vi "诊断标定3 - 副本.vi"(8 "CAN端口":u16(ring), 9 "设备索引号":u16(ring), 10 "CAN卡类型":u32(ring)=21) -> ()   [LabVIEW 2013] (continued)
                          n766 = Concatenate Strings("读取错误，代码： " ("字符串"), "0x" ("字符串"), w1225) -> (w1223:string)
                          n767 = One Button Dialog(message=w1223, button name ("OK")="是" ("按钮名称（“确定”）")) -> ()  [unwired: 1 out]
                        }
                      }
                      n768 = local write "消除"(FALSE ("消除")) -> ()
                      n769 = global write "EV05全局变量1.vi" "流控帧 2"(FALSE ("流控帧 2")) -> ()
                      n770 = local write "控制1"(FALSE ("控制1")) -> ()
                      n771 = global write "EV05全局变量1.vi" "写入超时"(TRUE ("写入超时")) -> ()
                    }
                  }
                }
              }
            }
          }
        }
      }
      frame Error {
      }
    }
  }
  n772 = while {
    tunnel: w36 -> [w1240]
    tunnel: w35 -> [w1239]
    tunnel: [w1238] -> w34
    tunnel: [w1237] -> w33
    tunnel: w23 -> [_]
    tunnel: w20 -> [_]
    stop <- w1236 stop-if-true
    n773 = event shown="[16] \"主板选项\": 鼠标按下" {
      selector: _ -> [_ _ _ _ _ _ _ _ _ _ _ _ _ _ _ _ _ _ _ _ _ _ _ _ _ _ _ _ _ _ _ _ _ _ _ _ _ _ _ _ _ _ _ _ _ _ _ _ _ _ _ _ _]
      dyn-events: _ -> [_ _ _ _ _ _ _ _ _ _ _ _ _ _ _ _ _ _ _ _ _ _ _ _ _ _ _ _ _ _ _ _ _ _ _ _ _ _ _ _ _ _ _ _ _ _ _ _ _ _ _ _ _]
      timeout: 200 -> [_ _ _ _ _ _ _ _ _ _ _ _ _ _ _ _ _ _ _ _ _ _ _ _ _ _ _ _ _ _ _ _ _ _ _ _ _ _ _ _ _ _ _ _ _ _ _ _ _ _ _ _ _]
      tunnel: [_ w1243 w1283 _ _ _ _ _ _ _ _ _ _ _ _ _ _ _ _ _ _ _ _ _ _ _ _ _ _ _ _ _ _ _ _ _ _ _ _ _ _ _ _ _ _ _ _ _ _ _ _ _ _] -> w1235
      tunnel: w1240 -> [w1242 w1246 w1282 _ w1323 w1334 w1345 w1356 w1367 w1378 w1389 w1400 w1411 w1422 w1433 w1444 w1460 w1998 w2420 w2445 w2473 w2576 w2649 w2662 w2672 w2718 _ _ w2768 w2835 w2902 w2969 w3036 w3103 w3170 w3238 w3306 w3373 w3440 w3510 w3521 w3560 w3600 w3640 w3680 w3718 w3778 w3813 w3849 w3882 w3952 w3985 w4018]
      tunnel: w1239 -> [w1241 w1245 w1281 _ w1322 w1333 w1344 w1355 w1366 w1377 w1388 w1399 w1410 w1421 w1432 w1443 w1459 w1997 w2419 w2444 w2472 w2575 w2647 w2660 w2671 w2717 _ _ w2767 w2834 w2901 w2968 w3035 w3102 w3169 w3237 w3305 w3372 w3439 w3508 w3520 w3559 w3599 w3639 w3679 w3717 w3777 w3812 w3848 w3881 w3951 w3984 w4017]
      tunnel: [w1242 w1246 w1282 _ w1323 w1334 w1345 w1356 w1367 w1378 w1389 w1400 w1411 w1422 w1433 w1444 w1460 w1998 w2420 w2445 w2473 w2576 w2648 w2661 w2672 w2718 _ _ w2768 w2835 w2902 w2969 w3036 w3103 w3170 w3238 w3306 w3373 w3440 w3509 w3519 w3558 w3598 w3638 w3678 w3718 w3776 w3811 w3847 w3880 w3950 w3983 w4016] -> w1238
      tunnel: [w1241 w1245 w1281 _ w1322 w1333 w1344 w1355 w1366 w1377 w1388 w1399 w1410 w1421 w1432 w1443 w1459 w1997 w2419 w2444 w2472 w2575 w2646 w2659 w2671 w2717 _ _ w2767 w2834 w2901 w2968 w3035 w3102 w3169 w3237 w3305 w3372 w3439 w3507 w3518 w3557 w3597 w3637 w3677 w3717 w3775 w3810 w3846 w3879 w3949 w3982 w4015] -> w1237
      tunnel: [_ _ _ _ _ _ _ _ _ _ _ _ _ _ _ _ _ _ _ _ _ _ _ _ _ _ _ _ _ _ _ _ _ _ _ _ _ _ _ _ w3518 w3557 w3597 w3637 w3677 _ w3775 w3810 w3846 w3879 w3949 w3982 w4015] -> w1234
      event Timeout {
        n774 = event-data() -> ()  [unwired: 3 out]
      }
      event "停止": Value Change {
        n775 = event-data() -> ("NewVal"=w1244:bool)  [unwired: 5 out]
        n776 = stacked-sequence {
          tunnel: w1244 -> [w1263 _]
          tunnel: [w1263 _] -> w1243
          frame #0 {
            n777 = global read "配置文件全局.vi" "诊断标定读取地址"() -> (w1247:path)
            n778 = call <vilib>:"Application Directory.vi"() -> ("Application Directory"=w1257:path)
            n779 = property class="VI"("FP.State"=T24."Hidden" ("前面板窗口:状态")) -> (reference out=w1259:refnum<vi>, error out=w1258:errorcluster)  [unwired: 2 in]
            n780 = Build Path(base path=w1257, name or relative path="config.ini" ("名称或相对路径")) -> (appended path=w1255:path)
            n781 = call <vilib>:"Open Config Data.vi"("configuration file path"=w1255) -> ("error out"=w1252:errorcluster, "refnum"=w1254:T25)  [unwired: 8 in, 1 out]
            n782 = local write "停止"(TRUE ("停止")) -> ()
            n783 = property class="VI"(reference=w1259, error in=w1258, "Front Panel.Open"=FALSE ("前面板窗口:打开")) -> ()  [unwired: 2 out]
            n784 = call-poly <vilib>:"Write Key.vi"("section"="总信息", "error in (no error)"=w1252, "value"=w1247, "key"="诊断标定读取地址" ("section"), "refnum"=w1254) -> ("error out"=w1251:errorcluster, "refnum out"=w1250:T25)  [unwired: 4 in, 1 out]
            n785 = call <vilib>:"Close Config Data.vi"("error in (no error)"=w1251, "refnum"=w1250) -> ("error out"=w1249:errorcluster)  [unwired: 8 in, 1 out]
            n786 = call <vilib>:"Clear Errors.vi"("error in (no error)"=w1249) -> ()  [unwired: 6 in, 1 out]
          }
          frame #1 {
            n787 = disable-structure shown="禁用" {
              frame Disabled {
                n788 = local read "设备索引号"() -> (w1269:u16)
                n789 = local read "CAN卡类型"() -> (w1270:u32)
                n790 = local read "CAN端口"() -> (w1268:u16)
                n791 = Build Array(7) -> (w1265:i32[])
                n792 = call "transmit-8.6.vi"("can卡类型"=w1270, "设备索引号"=w1269, "CAN端口"=w1268, "ID"=418398080, "SendType"=u8 0, "Data"=w1265) -> ()  [unwired: 3 in, 11 out]
              }
              frame Enabled {
                w1277 = u8 0 items=["Normal", "Listen Only"] ("工作方式")
                w1276 = u8 1 items=["Dual Filter", "Single Filter"] ("滤波方式")
                n793 = local read "设备索引号"() -> (w1272:u16)
                n794 = local read "CAN卡类型"() -> (w1271:u32)
                n795 = local read "CAN端口"() -> (w1273:u16)
                n796 = call "CAN_Init-8.6.vi"("CAN卡类型"=w1271, "设备索引号"=w1272, "CAN端口"=w1273, "操作类型"=enum16{"初始化CAN", "关闭CAN"}."初始化CAN", "滤波方式"=w1276, "Accept Code"=u32 0, "簇"=T21 {"打开CAN"=FALSE, "初始化CAN"=TRUE, "开始CAN"=TRUE, "重启"=FALSE, "关闭CAN"=FALSE}, "Mask Code"=u32 4294967295 ("Accept Code"), "工作方式"=w1277, "是否滤波"=FALSE) -> ()  [unwired: 4 in, 6 out]
              }
            }
          }
        }
      }
      event Panel Close? {
        n797 = event-data() -> ()  [unwired: 5 out]
        n798 = stacked-sequence {
          tunnel: [w1296 _] -> w1283
          frame #0 {
            w1296 = TRUE ("前面板窗口:打开")
            n799 = global read "配置文件全局.vi" "诊断标定读取地址"() -> (w1285:path)
            n800 = call <vilib>:"Application Directory.vi"() -> ("Application Directory"=w1295:path)
            n801 = property class="VI"("FP.State"=T24."Hidden" ("前面板窗口:状态")) -> (reference out=w1298:refnum<vi>, error out=w1297:errorcluster)  [unwired: 2 in]
            n802 = Build Path(base path=w1295, name or relative path="config.ini" ("名称或相对路径")) -> (appended path=w1293:path)
            n803 = call <vilib>:"Open Config Data.vi"("configuration file path"=w1293) -> ("error out"=w1290:errorcluster, "refnum"=w1292:T25)  [unwired: 8 in, 1 out]
            n804 = property class="VI"(reference=w1298, error in=w1297, "Front Panel.Open"=FALSE ("前面板窗口:打开")) -> ()  [unwired: 2 out]
            n805 = call-poly <vilib>:"Write Key.vi"("section"="总信息", "error in (no error)"=w1290, "value"=w1285, "key"="诊断标定读取地址" ("section"), "refnum"=w1292) -> ("error out"=w1289:errorcluster, "refnum out"=w1288:T25)  [unwired: 4 in, 1 out]
            n806 = call <vilib>:"Close Config Data.vi"("error in (no error)"=w1289, "refnum"=w1288) -> ("error out"=w1287:errorcluster)  [unwired: 8 in, 1 out]
            n807 = call <vilib>:"Clear Errors.vi"("error in (no error)"=w1287) -> ()  [unwired: 6 in, 1 out]
            n808 = local write "强制终止读写标记"(TRUE ("强制终止读写标记")) -> ()
            n809 = local write "停止"(w1296) -> ()
          }
          frame #1 {
            w1304 = u8 0 items=["Normal", "Listen Only"] ("工作方式")
            w1305 = u8 1 items=["Dual Filter", "Single Filter"] ("滤波方式")
            n810 = local read "设备索引号"() -> (w1309:u16)
            n811 = local read "CAN卡类型"() -> (w1310:u32)
            n812 = local read "CAN端口"() -> (w1308:u16)
            n813 = call "CAN_Init-8.6.vi"("CAN卡类型"=w1310, "设备索引号"=w1309, "CAN端口"=w1308, "操作类型"=enum16{"初始化CAN", "关闭CAN"}."初始化CAN", "滤波方式"=w1305, "Accept Code"=u32 0, "簇"=T21 {"打开CAN"=FALSE, "初始化CAN"=TRUE, "开始CAN"=TRUE, "重启"=FALSE, "关闭CAN"=FALSE}, "Mask Code"=u32 4294967295 ("Accept Code"), "工作方式"=w1304, "是否滤波"=FALSE) -> ()  [unwired: 4 in, 6 out]
          }
        }
        n814 = event-data("Discard?"=w1283) -> ()  [unwired: 1 in, 1 out]
      }
      event "终止读写按钮": Value Change {
        n815 = event-data() -> ("NewVal"=w1311:bool)  [unwired: 6 out]
        n816 = case shown="真" w1311 {
          frame False {
          }
          frame True {
            n817 = local write "强制终止读写标记"(TRUE ("强制终止读写标记")) -> ()
          }
        }
      }
      event "1": Value Change {
        w1320 = FALSE ("1")
        n818 = event-data() -> ()  [unwired: 7 out]
        n819 = local write "主板2"(T8."项目信息" ("主从板")) -> ()
        n820 = Not(x=w1320) -> (.not. x?=w1319:bool)
        n821 = local write "1"(w1319) -> ()
        n822 = local write "1 2"(w1320) -> ()
        n823 = local write "1 3"(w1320) -> ()
        n824 = local write "1 4"(w1320) -> ()
        n825 = local write "1 5"(w1320) -> ()
        n826 = local write "1 11"(w1320) -> ()
        n827 = global read "功能码全局.vi" "主板监控2"() -> (w1318:bool[])
        n828 = Index Array(array=w1318, index=6 ("索引")) -> (element=w1313:bool)
        n829 = Select(t=0, s=w1313, f=1) -> (s? t:f=w1314:i32)
        n830 = property on="项目信息" class="Tbl (严格)"("Disabled"=w1314) -> ()  [unwired: 2 in, 2 out]
        n831 = property on="电池实际容量(A)" class="DigNum (严格)"("Disabled"=w1314) -> ()  [unwired: 2 in, 2 out]
        n832 = property on="使用者" class="DigNum (严格)"("Disabled"=w1314) -> ()  [unwired: 2 in, 2 out]
        n833 = property on="SOH(%)" class="DigNum (严格)"("Disabled"=w1314) -> ()  [unwired: 2 in, 2 out]
        n834 = property on="电池额定容量(A)" class="DigNum (严格)"("Disabled"=w1314) -> ()  [unwired: 2 in, 2 out]
        n835 = property on="SOC(%)" class="DigNum (严格)"("Disabled"=w1314) -> ()  [unwired: 2 in, 2 out]
        n836 = property on="项目信息2" class="Clust (严格)"("DisabledEnum"=w1314) -> ()  [unwired: 2 in, 2 out]
        n837 = property on="系统时钟" class="Str"("Disabled"=w1314) -> ()  [unwired: 2 in, 2 out]
        n838 = property on="配置文件版本" class="Str"("Disabled"=w1314) -> ()  [unwired: 2 in, 2 out]
        n839 = property on="车架(牌)号" class="Str"("Disabled"=w1314) -> ()  [unwired: 2 in, 2 out]
        n840 = property on="产品编号" class="Str"("Disabled"=w1314) -> ()  [unwired: 2 in, 2 out]
      }
      event "1 2": Value Change {
        w1331 = FALSE ("1")
        n841 = event-data() -> ()  [unwired: 7 out]
        n842 = local write "主板2"(T8."一级故障阀值" ("主从板")) -> ()
        n843 = Not(x=w1331) -> (.not. x?=w1330:bool)
        n844 = local write "1"(w1331) -> ()
        n845 = local write "1 2"(w1330) -> ()
        n846 = local write "1 3"(w1331) -> ()
        n847 = local write "1 4"(w1331) -> ()
        n848 = local write "1 5"(w1331) -> ()
        n849 = local write "1 11"(w1331) -> ()
        n850 = global read "功能码全局.vi" "主板监控2"() -> (w1329:bool[])
        n851 = Index Array(array=w1329, index=6 ("索引")) -> (element=w1324:bool)
        n852 = Select(t=0, s=w1324, f=1) -> (s? t:f=w1327:i32)
        n853 = property on="一级故障" class="Clust (严格)"("DisabledEnum"=w1327) -> ()  [unwired: 2 in, 2 out]
      }
      event "1 3": Value Change {
        w1342 = FALSE ("1")
        n854 = event-data() -> ()  [unwired: 7 out]
        n855 = local write "主板2"(T8."二级故障阀值" ("主从板")) -> ()
        n856 = Not(x=w1342) -> (.not. x?=w1341:bool)
        n857 = local write "1"(w1342) -> ()
        n858 = local write "1 2"(w1342) -> ()
        n859 = local write "1 3"(w1341) -> ()
        n860 = local write "1 4"(w1342) -> ()
        n861 = local write "1 5"(w1342) -> ()
        n862 = local write "1 11"(w1342) -> ()
        n863 = global read "功能码全局.vi" "主板监控2"() -> (w1340:bool[])
        n864 = Index Array(array=w1340, index=6 ("索引")) -> (element=w1336:bool)
        n865 = Select(t=0, s=w1336, f=1) -> (s? t:f=w1335:i32)
        n866 = property on="一级故障 2" class="Clust (严格)"("DisabledEnum"=w1335) -> ()  [unwired: 2 in, 2 out]
      }
      event "1 4": Value Change {
        w1353 = FALSE ("1")
        n867 = event-data() -> ()  [unwired: 7 out]
        n868 = local write "主板2"(T8."三级故障阀值" ("主从板")) -> ()
        n869 = Not(x=w1353) -> (.not. x?=w1352:bool)
        n870 = local write "1"(w1353) -> ()
        n871 = local write "1 2"(w1353) -> ()
        n872 = local write "1 3"(w1353) -> ()
        n873 = local write "1 4"(w1352) -> ()
        n874 = local write "1 5"(w1353) -> ()
        n875 = local write "1 11"(w1353) -> ()
        n876 = global read "功能码全局.vi" "主板监控2"() -> (w1351:bool[])
        n877 = Index Array(array=w1351, index=6 ("索引")) -> (element=w1346:bool)
        n878 = Select(t=0, s=w1346, f=1) -> (s? t:f=w1349:i32)
        n879 = property on="一级故障 3" class="Clust (严格)"("DisabledEnum"=w1349) -> ()  [unwired: 2 in, 2 out]
      }
      event "1 5": Value Change {
        w1364 = FALSE ("1")
        n880 = event-data() -> ()  [unwired: 7 out]
        n881 = local write "主板2"(T8."控制参数" ("主从板")) -> ()
        n882 = Not(x=w1364) -> (.not. x?=w1363:bool)
        n883 = local write "1"(w1364) -> ()
        n884 = local write "1 2"(w1364) -> ()
        n885 = local write "1 3"(w1364) -> ()
        n886 = local write "1 4"(w1364) -> ()
        n887 = local write "1 5"(w1363) -> ()
        n888 = local write "1 11"(w1364) -> ()
        n889 = global read "功能码全局.vi" "主板监控2"() -> (w1360:bool[])
        n890 = Index Array(array=w1360, index=6 ("索引")) -> (element=w1358:bool)
        n891 = Select(t=0, s=w1358, f=1) -> (s? t:f=w1357:i32)
        n892 = property on="风机开启温度" class="DigNum (严格)"("Disabled"=w1357) -> ()  [unwired: 2 in, 2 out]
        n893 = property on="风机关闭温度" class="DigNum (严格)"("Disabled"=w1357) -> ()  [unwired: 2 in, 2 out]
        n894 = property on="加热开启温度" class="DigNum (严格)"("Disabled"=w1357) -> ()  [unwired: 2 in, 2 out]
        n895 = property on="加热关闭温度" class="DigNum (严格)"("Disabled"=w1357) -> ()  [unwired: 2 in, 2 out]
        n896 = property on="风机开启温差" class="DigNum (严格)"("Disabled"=w1357) -> ()  [unwired: 2 in, 2 out]
        n897 = property on="风机关闭温差" class="DigNum (严格)"("Disabled"=w1357) -> ()  [unwired: 2 in, 2 out]
        n898 = property on="加热控制参数" class="Clust (严格)"("DisabledEnum"=w1357) -> ()  [unwired: 2 in, 2 out]
        n899 = property on="最大允许总电压" class="DigNum (严格)"("Disabled"=w1357) -> ()  [unwired: 2 in, 2 out]
        n900 = property on="最大允许充电温度" class="DigNum (严格)"("Disabled"=w1357) -> ()  [unwired: 2 in, 2 out]
        n901 = property on="最小允许充电温度" class="DigNum (严格)"("Disabled"=w1357) -> ()  [unwired: 2 in, 2 out]
        n902 = property on="电流步长" class="DigNum (严格)"("Disabled"=w1357) -> ()  [unwired: 2 in, 2 out]
        n903 = property on="最大允许单体电压" class="DigNum (严格)"("Disabled"=w1357) -> ()  [unwired: 2 in, 2 out]
        n904 = property on="最小允许单体电压" class="DigNum (严格)"("Disabled"=w1357) -> ()  [unwired: 2 in, 2 out]
        n905 = property on="最大允许充电电流" class="DigNum (严格)"("Disabled"=w1357) -> ()  [unwired: 2 in, 2 out]
        n906 = property on="最小允许充电电流" class="DigNum (严格)"("Disabled"=w1357) -> ()  [unwired: 2 in, 2 out]
      }
      event "1 11": Value Change {
        w1375 = FALSE ("1")
        n907 = event-data() -> ()  [unwired: 7 out]
        n908 = local write "主板2"(T8."电池信息" ("主从板")) -> ()
        n909 = Not(x=w1375) -> (.not. x?=w1374:bool)
        n910 = local write "1"(w1375) -> ()
        n911 = local write "1 2"(w1375) -> ()
        n912 = local write "1 3"(w1375) -> ()
        n913 = local write "1 4"(w1375) -> ()
        n914 = local write "1 5"(w1375) -> ()
        n915 = local write "1 11"(w1374) -> ()
        n916 = global read "功能码全局.vi" "主板监控2"() -> (w1370:bool[])
        n917 = Index Array(array=w1370, index=6 ("索引")) -> (element=w1368:bool)
        n918 = Select(t=0, s=w1368, f=1) -> (s? t:f=w1371:i32)
        n919 = property on="电池串联" class="DigNum (严格)"("Disabled"=w1371) -> ()  [unwired: 2 in, 2 out]
        n920 = property on="电池并联" class="DigNum (严格)"("Disabled"=w1371) -> ()  [unwired: 2 in, 2 out]
        n921 = property on="电池包额定容量" class="DigNum (严格)"("Disabled"=w1371) -> ()  [unwired: 2 in, 2 out]
        n922 = property on="电池包额定能量(kWh)" class="DigNum (严格)"("Disabled"=w1371) -> ()  [unwired: 2 in, 2 out]
        n923 = property on="电池包额定总电压" class="DigNum (严格)"("Disabled"=w1371) -> ()  [unwired: 2 in, 2 out]
        n924 = property on="实际容量" class="DigNum (严格)"("Disabled"=w1371) -> ()  [unwired: 2 in, 2 out]
        n925 = property on="电池包组号" class="Str"("Disabled"=w1371) -> ()  [unwired: 2 in, 2 out]
        n926 = property on="电池生产日期" class="Str"("Disabled"=w1371) -> ()  [unwired: 2 in, 2 out]
        n927 = property on="电池厂家" class="Str"("Disabled"=w1371) -> ()  [unwired: 2 in, 2 out]
        n928 = property on="电池类型" class="Str"("Disabled"=w1371) -> ()  [unwired: 2 in, 2 out]
        n929 = property on="累计充电总安时" class="DigNum (严格)"("Disabled"=w1371) -> ()  [unwired: 2 in, 2 out]
        n930 = property on="累计放电总安时" class="DigNum (严格)"("Disabled"=w1371) -> ()  [unwired: 2 in, 2 out]
        n931 = property on="电池放空次数" class="DigNum (严格)"("Disabled"=w1371) -> ()  [unwired: 2 in, 2 out]
        n932 = property on="电池充满次数" class="DigNum (严格)"("Disabled"=w1371) -> ()  [unwired: 2 in, 2 out]
        n933 = property on="电池充电次数" class="DigNum (严格)"("Disabled"=w1371) -> ()  [unwired: 2 in, 2 out]
        n934 = property on="电池信息" class="Clust (严格)"("DisabledEnum"=w1371) -> ()  [unwired: 2 in, 2 out]
      }
      event "1 6": Value Change {
        w1386 = FALSE ("1 6")
        n935 = event-data() -> ()  [unwired: 7 out]
        n936 = local write "等级 2"(T19."从板信息" ("等级 2")) -> ()
        n937 = global read "功能码全局.vi" "主板监控2"() -> (w1381:bool[])
        n938 = Not(x=w1386) -> (.not. x?=w1385:bool)
        n939 = local write "1 6"(w1385) -> ()
        n940 = local write "1 7"(w1386) -> ()
        n941 = local write "1 8"(w1386) -> ()
        n942 = local write "1 9"(w1386) -> ()
        n943 = local write "1 10"(w1386) -> ()
        n944 = Index Array(array=w1381, index=6 ("索引")) -> (element=w1379:bool)
        n945 = Select(t=0, s=w1379, f=1) -> (s? t:f=w1382:i32)
        n946 = property on="项目信息 2" class="Tbl (严格)"("Disabled"=w1382) -> ()  [unwired: 2 in, 2 out]
        n947 = property on="加热控制参数" class="Clust (严格)"("Disabled"=w1382) -> ()  [unwired: 2 in, 2 out]
      }
      event "1 7": Value Change {
        w1397 = FALSE ("1 6")
        n948 = event-data() -> ()  [unwired: 7 out]
        n949 = global read "功能码全局.vi" "主板监控2"() -> (w1395:bool[])
        n950 = Index Array(array=w1395, index=6 ("索引")) -> (element=w1390:bool)
        n951 = local write "等级 2"(T19."一级故障阀值" ("等级 2")) -> ()
        n952 = Select(t=0, s=w1390, f=1) -> (s? t:f=w1391:i32)
        n953 = property on="一级故障 6" class="Clust (严格)"("DisabledEnum"=w1391) -> ()  [unwired: 2 in, 2 out]
        n954 = Not(x=w1397) -> (.not. x?=w1396:bool)
        n955 = local write "1 6"(w1397) -> ()
        n956 = local write "1 7"(w1396) -> ()
        n957 = local write "1 8"(w1397) -> ()
        n958 = local write "1 9"(w1397) -> ()
        n959 = local write "1 10"(w1397) -> ()
      }
      event "1 8": Value Change {
        w1408 = FALSE ("1 6")
        n960 = event-data() -> ()  [unwired: 7 out]
        n961 = global read "功能码全局.vi" "主板监控2"() -> (w1406:bool[])
        n962 = Index Array(array=w1406, index=6 ("索引")) -> (element=w1401:bool)
        n963 = local write "等级 2"(T19."二级故障阀值" ("等级 2")) -> ()
        n964 = Select(t=0, s=w1401, f=1) -> (s? t:f=w1402:i32)
        n965 = Not(x=w1408) -> (.not. x?=w1407:bool)
        n966 = property on="一级故障 7" class="Clust (严格)"("DisabledEnum"=w1402) -> ()  [unwired: 2 in, 2 out]
        n967 = local write "1 6"(w1408) -> ()
        n968 = local write "1 7"(w1408) -> ()
        n969 = local write "1 8"(w1407) -> ()
        n970 = local write "1 9"(w1408) -> ()
        n971 = local write "1 10"(w1408) -> ()
      }
      event "1 9": Value Change {
        w1419 = FALSE ("1 6")
        n972 = event-data() -> ()  [unwired: 7 out]
        n973 = global read "功能码全局.vi" "主板监控2"() -> (w1417:bool[])
        n974 = Index Array(array=w1417, index=6 ("索引")) -> (element=w1412:bool)
        n975 = Select(t=0, s=w1412, f=1) -> (s? t:f=w1413:i32)
        n976 = local write "等级 2"(T19."三级故障阀值" ("等级 2")) -> ()
        n977 = property on="一级故障 8" class="Clust (严格)"("DisabledEnum"=w1413) -> ()  [unwired: 2 in, 2 out]
        n978 = Not(x=w1419) -> (.not. x?=w1418:bool)
        n979 = local write "1 6"(w1419) -> ()
        n980 = local write "1 7"(w1419) -> ()
        n981 = local write "1 8"(w1419) -> ()
        n982 = local write "1 9"(w1418) -> ()
        n983 = local write "1 10"(w1419) -> ()
      }
      event "1 10": Value Change {
        w1430 = FALSE ("1 6")
        n984 = event-data() -> ()  [unwired: 7 out]
        n985 = global read "功能码全局.vi" "主板监控2"() -> (w1428:bool[])
        n986 = Index Array(array=w1428, index=6 ("索引")) -> (element=w1423:bool)
        n987 = Select(t=0, s=w1423, f=1) -> (s? t:f=w1424:i32)
        n988 = local write "等级 2"(T19."快换参数" ("等级 2")) -> ()
        n989 = property on="电池组信息" class="Clust (严格)"("Disabled"=w1424) -> ()  [unwired: 2 in, 2 out]
        n990 = Not(x=w1430) -> (.not. x?=w1429:bool)
        n991 = local write "1 6"(w1430) -> ()
        n992 = local write "1 7"(w1430) -> ()
        n993 = local write "1 8"(w1430) -> ()
        n994 = local write "1 9"(w1430) -> ()
        n995 = local write "1 10"(w1429) -> ()
      }
      event "1 12": Value Change {
        w1435 = FALSE ("1 6")
        n996 = event-data() -> ()  [unwired: 7 out]
        n997 = global read "功能码全局.vi" "主板监控2"() -> (w1442:bool[])
        n998 = Index Array(array=w1442, index=6 ("索引")) -> (element=w1438:bool)
        n999 = Select(t=0, s=w1438, f=1) -> (s? t:f=w1434:i32)
        n1000 = local write "等级 2"(T14."均衡参数" ("等级 2")) -> ()
        n1001 = property on="均衡参数" class="Clust (严格)"("DisabledEnum"=w1434) -> ()  [unwired: 2 in, 2 out]
        n1002 = Not(x=w1435) -> (.not. x?=w1436:bool)
        n1003 = local write "1 12"(w1436) -> ()
        n1004 = local write "1 6"(w1435) -> ()
        n1005 = local write "1 7"(w1435) -> ()
        n1006 = local write "1 8"(w1435) -> ()
        n1007 = local write "1 9"(w1435) -> ()
        n1008 = local write "1 10"(w1435) -> ()
      }
      event "主板选项": Mouse Down {
        n1009 = event-data() -> ("CtlRef"=w1458:refnum<vi>)  [unwired: 8 out]
        n1010 = global read "功能码全局.vi" "主板监控2"() -> (w1447:bool[])
        n1011 = property class="Tree (严格)"(reference=w1458) -> ("Value"=w1450:string)  [unwired: 1 in, 2 out]
        n1012 = Index Array(array=w1447, index=6 ("索引")) -> (element=w1445:bool)
        n1013 = case shown="\"二维码\"" w1450 {
          tunnel: [T8."项目信息" ("主从板") T8."项目信息" ("主从板") T8."项目信息" ("主从板") T8."项目信息" ("主从板") T8."项目信息" ("主从板") T8."项目信息" ("主从板") T8."项目信息" ("主从板") T8."项目信息" ("主从板") T8."项目信息" ("主从板") T8."项目信息" ("主从板") T8."项目信息" ("主从板") T8."项目信息" ("主从板") T8."项目信息" ("主从板") T8."项目信息" ("主从板") T8."项目信息" ("主从板") T8."项目信息" ("主从板") T8."二级故障阀值" ("主从板") T8."三级故障阀值" ("主从板") T8."一级故障阀值" ("主从板") T8."控制参数" ("主从板") T8."控制参数" ("主从板") T8."电池信息" ("主从板") T8."电池信息" ("主从板") T8."电池信息" ("主从板") T8."电池信息" ("主从板") T8."电池信息" ("主从板") T8."项目信息" ("主从板")] -> w1457
          tunnel: [w1468 w1475 w1490 w1505 w1522 w1562 w1596 w1643 w1681 w1731 w1766 w1780 w1795 w1810 w1825 w1839 w1852 w1866 w1879 w1893 w1907 w1920 w1934 w1948 w1962 w1976 w1980] -> w1456
          tunnel: [w1469 w1476 w1491 w1506 w1523 w1563 w1597 w1644 w1682 w1732 w1767 w1781 w1796 w1811 w1826 w1840 w1852 w1866 w1878 w1893 w1907 w1920 w1934 w1948 w1962 w1976 w1981] -> w1455
          tunnel: [w1469 w1476 w1491 w1506 w1523 w1563 w1597 w1644 w1682 w1732 w1767 w1781 w1796 w1811 w1826 w1840 w1853 w1866 w1879 w1893 w1907 w1920 w1934 w1948 w1962 w1976 w1981] -> w1454
          tunnel: [w1469 w1476 w1491 w1506 w1523 w1563 w1597 w1644 w1682 w1732 w1767 w1781 w1796 w1811 w1826 w1840 w1852 w1865 w1879 w1893 w1907 w1920 w1934 w1948 w1962 w1976 w1981] -> w1453
          tunnel: [w1469 w1476 w1491 w1506 w1523 w1563 w1597 w1644 w1682 w1732 w1767 w1781 w1796 w1811 w1826 w1840 w1852 w1866 w1879 w1892 w1906 w1920 w1934 w1948 w1962 w1976 w1981] -> w1452
          tunnel: [w1469 w1476 w1491 w1506 w1523 w1563 w1597 w1644 w1682 w1732 w1767 w1781 w1796 w1811 w1826 w1840 w1852 w1866 w1879 w1893 w1907 w1919 w1933 w1947 w1961 w1975 w1981] -> w1451
          tunnel: [w1461 FALSE w1486 w1501 w1514 w1554 w1587 w1634 w1673 w1724 w1761 w1775 w1789 w1803 w1818 w1834 w1848 w1861 w1874 w1888 w1901 w1915 w1928 w1942 w1956 w1970 FALSE] -> w1449
          tunnel: [w1461 TRUE w1483 w1498 w1513 w1553 w1588 w1635 w1672 w1723 w1760 w1774 w1788 w1804 w1819 w1833 w1847 w1860 w1873 w1887 w1900 w1914 w1927 w1941 w1955 w1969 FALSE] -> w1448
          tunnel: w1445 -> [w1466 _ w1480 w1495 w1510 w1549 w1584 w1631 w1669 w1721 w1757 w1771 w1785 w1800 w1815 w1830 w1844 w1857 w1870 w1884 w1897 w1911 w1924 w1938 w1952 w1966 _]
          frame "项目信息" {
            w1469 = FALSE
            n1014 = Select(t=0, s=w1466, f=1) -> (s? t:f=w1464:i32)
            n1015 = property on="项目信息" class="Tbl (严格)"("Disabled"=w1464) -> ()  [unwired: 2 in, 2 out]
            n1016 = property on="电池实际容量(A)" class="DigNum (严格)"("Disabled"=w1464) -> ()  [unwired: 2 in, 2 out]
            n1017 = property on="使用者" class="DigNum (严格)"("Disabled"=w1464) -> ()  [unwired: 2 in, 2 out]
            n1018 = property on="SOH(%)" class="DigNum (严格)"("Disabled"=w1464) -> ()  [unwired: 2 in, 2 out]
            n1019 = property on="从板个数" class="DigNum (严格)"("NumText.BGColor"=u32 6618880) -> ()  [unwired: 2 in, 2 out]
            n1020 = property on="电池额定容量(A)" class="DigNum (严格)"("Disabled"=w1464) -> ()  [unwired: 2 in, 2 out]
            n1021 = property on="SOC(%)" class="DigNum (严格)"("Disabled"=w1464) -> ()  [unwired: 2 in, 2 out]
            n1022 = property on="项目信息2" class="Clust (严格)"("DisabledEnum"=w1464) -> ()  [unwired: 2 in, 2 out]
            n1023 = property on="系统时钟" class="Str"("Disabled"=w1464) -> ()  [unwired: 2 in, 2 out]
            n1024 = property on="配置文件版本" class="Str"("Disabled"=w1464) -> ()  [unwired: 2 in, 2 out]
            n1025 = property on="车架(牌)号" class="Str"("Disabled"=w1464) -> ()  [unwired: 2 in, 2 out]
            n1026 = property on="产品编号" class="Str"("Disabled"=w1464) -> ()  [unwired: 2 in, 2 out]
            n1027 = local read "项目信息结果"() -> (w1462:bool)
            n1028 = Not(x=w1462) -> (.not. x?=w1461:bool)
            n1029 = Not(x=w1469) -> (.not. x?=w1468:bool)
          }
          frame "校正时钟" {
            w1472 = 2
            w1476 = FALSE
            n1030 = property on="从板个数" class="DigNum (严格)"("NumText.BGColor"=u32 13816530) -> ()  [unwired: 2 in, 2 out]
            n1031 = property on="项目信息" class="Tbl (严格)"("Disabled"=w1472) -> ()  [unwired: 2 in, 2 out]
            n1032 = property on="电池实际容量(A)" class="DigNum (严格)"("Disabled"=w1472) -> ()  [unwired: 2 in, 2 out]
            n1033 = property on="使用者" class="DigNum (严格)"("Disabled"=w1472) -> ()  [unwired: 2 in, 2 out]
            n1034 = property on="SOH(%)" class="DigNum (严格)"("Disabled"=w1472) -> ()  [unwired: 2 in, 2 out]
            n1035 = property on="电池额定容量(A)" class="DigNum (严格)"("Disabled"=w1472) -> ()  [unwired: 2 in, 2 out]
            n1036 = property on="SOC(%)" class="DigNum (严格)"("Disabled"=w1472) -> ()  [unwired: 2 in, 2 out]
            n1037 = property on="系统时钟" class="Str"("Disabled"=w1472) -> ()  [unwired: 2 in, 2 out]
            n1038 = property on="配置文件版本" class="Str"("Disabled"=w1472) -> ()  [unwired: 2 in, 2 out]
            n1039 = property on="车架(牌)号" class="Str"("Disabled"=w1472) -> ()  [unwired: 2 in, 2 out]
            n1040 = property on="项目信息2" class="Clust (严格)"("DisabledEnum"=w1472) -> ()  [unwired: 2 in, 2 out]
            n1041 = property on="产品编号" class="Str"("Disabled"=w1472) -> ()  [unwired: 2 in, 2 out]
            n1042 = Not(x=w1476) -> (.not. x?=w1475:bool)
          }
          frame "产品编号" {
            w1489 = 2
            w1491 = FALSE
            n1043 = property on="项目信息" class="Tbl (严格)"("Disabled"=w1489) -> ()  [unwired: 2 in, 2 out]
            n1044 = property on="电池实际容量(A)" class="DigNum (严格)"("Disabled"=w1489) -> ()  [unwired: 2 in, 2 out]
            n1045 = property on="使用者" class="DigNum (严格)"("Disabled"=w1489) -> ()  [unwired: 2 in, 2 out]
            n1046 = Select(t=0, s=w1480, f=1) -> (s? t:f=w1479:i32)
            n1047 = property on="SOH(%)" class="DigNum (严格)"("Disabled"=w1489) -> ()  [unwired: 2 in, 2 out]
            n1048 = property on="电池额定容量(A)" class="DigNum (严格)"("Disabled"=w1489) -> ()  [unwired: 2 in, 2 out]
            n1049 = property on="SOC(%)" class="DigNum (严格)"("Disabled"=w1489) -> ()  [unwired: 2 in, 2 out]
            n1050 = property on="产品编号" class="Str"("Disabled"=w1479) -> ()  [unwired: 2 in, 2 out]
            n1051 = property on="项目信息2" class="Clust (严格)"("DisabledEnum"=w1479) -> ()  [unwired: 2 in, 2 out]
            n1052 = property on="系统时钟" class="Str"("Disabled"=w1489) -> ()  [unwired: 2 in, 2 out]
            n1053 = property on="配置文件版本" class="Str"("Disabled"=w1489) -> ()  [unwired: 2 in, 2 out]
            n1054 = property on="车架(牌)号" class="Str"("Disabled"=w1489) -> ()  [unwired: 2 in, 2 out]
            n1055 = property on="从板个数" class="DigNum (严格)"("NumText.BGColor"=u32 13816530) -> ()  [unwired: 2 in, 2 out]
            n1056 = global read "功能码全局.vi" "主板项目信息5"() -> (w1487:bool[])
            n1057 = global read "功能码全局.vi" "主板项目信息6"() -> (w1484:bool[])
            n1058 = Index Array(array=w1487, index=0 ("索引")) -> (element=w1486:bool)
            n1059 = Index Array(array=w1484, index=1 ("索引")) -> (element=w1483:bool)
            n1060 = Not(x=w1491) -> (.not. x?=w1490:bool)
          }
          frame "二维码" {
            w1504 = 2
            w1506 = FALSE
            n1061 = property on="项目信息" class="Tbl (严格)"("Disabled"=w1504) -> ()  [unwired: 2 in, 2 out]
            n1062 = property on="电池实际容量(A)" class="DigNum (严格)"("Disabled"=w1504) -> ()  [unwired: 2 in, 2 out]
            n1063 = property on="使用者" class="DigNum (严格)"("Disabled"=w1504) -> ()  [unwired: 2 in, 2 out]
            n1064 = Select(t=0, s=w1495, f=1) -> (s? t:f=w1494:i32)
            n1065 = property on="SOH(%)" class="DigNum (严格)"("Disabled"=w1504) -> ()  [unwired: 2 in, 2 out]
            n1066 = property on="电池额定容量(A)" class="DigNum (严格)"("Disabled"=w1504) -> ()  [unwired: 2 in, 2 out]
            n1067 = property on="SOC(%)" class="DigNum (严格)"("Disabled"=w1504) -> ()  [unwired: 2 in, 2 out]
            n1068 = property on="产品编号" class="Str"("Disabled"=w1494) -> ()  [unwired: 2 in, 2 out]
            n1069 = property on="项目信息2" class="Clust (严格)"("DisabledEnum"=w1494) -> ()  [unwired: 2 in, 2 out]
            n1070 = property on="系统时钟" class="Str"("Disabled"=w1504) -> ()  [unwired: 2 in, 2 out]
            n1071 = property on="配置文件版本" class="Str"("Disabled"=w1504) -> ()  [unwired: 2 in, 2 out]
            n1072 = property on="车架(牌)号" class="Str"("Disabled"=w1504) -> ()  [unwired: 2 in, 2 out]
            n1073 = property on="从板个数" class="DigNum (严格)"("NumText.BGColor"=u32 13816530) -> ()  [unwired: 2 in, 2 out]
            n1074 = global read "功能码全局.vi" "主板项目信息5"() -> (w1502:bool[])
            n1075 = global read "功能码全局.vi" "主板项目信息6"() -> (w1499:bool[])
            n1076 = Index Array(array=w1502, index=0 ("索引")) -> (element=w1501:bool)
            n1077 = Index Array(array=w1499, index=1 ("索引")) -> (element=w1498:bool)
            n1078 = Not(x=w1506) -> (.not. x?=w1505:bool)
          }
          frame "电压个数" {
            w1521 = 2
            w1523 = FALSE
            n1079 = local read "从板个数"() -> (w1520:dbl)
            n1080 = property on="从板个数" class="DigNum (严格)"("NumText.BGColor"=u32 6618880) -> ()  [unwired: 2 in, 2 out]
            n1081 = property on="电池实际容量(A)" class="DigNum (严格)"("Disabled"=w1521) -> ()  [unwired: 2 in, 2 out]
            n1082 = property on="使用者" class="DigNum (严格)"("Disabled"=w1521) -> ()  [unwired: 2 in, 2 out]
            n1083 = property on="SOH(%)" class="DigNum (严格)"("Disabled"=w1521) -> ()  [unwired: 2 in, 2 out]
            n1084 = property on="电池额定容量(A)" class="DigNum (严格)"("Disabled"=w1521) -> ()  [unwired: 2 in, 2 out]
            n1085 = property on="SOC(%)" class="DigNum (严格)"("Disabled"=w1521) -> ()  [unwired: 2 in, 2 out]
            n1086 = property on="系统时钟" class="Str"("Disabled"=w1521) -> ()  [unwired: 2 in, 2 out]
            n1087 = property on="配置文件版本" class="Str"("Disabled"=w1521) -> ()  [unwired: 2 in, 2 out]
            n1088 = property on="车架(牌)号" class="Str"("Disabled"=w1521) -> ()  [unwired: 2 in, 2 out]
            n1089 = property on="产品编号" class="Str"("Disabled"=w1521) -> ()  [unwired: 2 in, 2 out]
            n1090 = Select(t=0, s=w1510, f=1) -> (s? t:f=w1509:i32)
            n1091 = control-ref of="项目信息"() -> (w1519:refnum<vi>)
            n1092 = stacked-sequence {
              tunnel: w1520 -> [_ w1530 w1540]
              tunnel: w1519 -> [w1525 w1529 w1541]
              frame #0 {
                w1526 = 0
                n1093 = Bundle(w1526, w1526) -> (w1528:cluster{i32, i32})  [unwired: 1 out]
                n1094 = property class="Tbl (严格)"(reference=w1525, "Index Values"=w1528) -> (error out=w1527:errorcluster)  [unwired: 1 in, 1 out]
                n1095 = call <vilib>:"Clear Errors.vi"("error in (no error)"=w1527) -> ()  [unwired: 7 out]
              }
              frame #1 {
                n1096 = for {
                  N: 10 -> [_]
                  tunnel: w1529 -> [w1539]
                  tunnel: w1530 -> [w1534]
                  i -> [w1533]
                  n1097 = Compound Arithmetic op=ADD(0.0 ("值"), w1534, w1533) -> (w1536:dbl)
                  n1098 = Bundle(w1536, 0) -> (w1538:cluster{dbl, i32})  [unwired: 1 out]
                  n1099 = property class="Tbl (严格)"(reference=w1539, "Active Cell"=w1538, "Cell BG Color"=u32 16448250) -> ()  [unwired: 1 in, 2 out]
                }
              }
              frame #2 {
                n1100 = for {
                  N: w1540 -> [_]
                  tunnel: w1541 -> [w1542]
                  i -> [w1543]
                  n1101 = Bundle(w1543, 0) -> (w1547:cluster{i32, i32})  [unwired: 1 out]
                  n1102 = property class="Tbl (严格)"(reference=w1542, "Active Cell"=w1547, "Cell BG Color"=u32 6618880) -> (error out=w1544:errorcluster)  [unwired: 1 in, 1 out]
                  n1103 = call <vilib>:"Clear Errors.vi"("error in (no error)"=w1544) -> ()  [unwired: 7 out]
                }
              }
            }
            n1104 = property on="项目信息" class="Tbl (严格)"("Disabled"=w1509) -> ()  [unwired: 2 in, 2 out]
            n1105 = global read "功能码全局.vi" "主板项目信息5"() -> (w1517:bool[])
            n1106 = global read "功能码全局.vi" "主板项目信息6"() -> (w1515:bool[])
            n1107 = Index Array(array=w1517, index=1 ("索引")) -> (element=w1514:bool)
            n1108 = Index Array(array=w1515, index=2 ("索引")) -> (element=w1513:bool)
            n1109 = Not(x=w1523) -> (.not. x?=w1522:bool)
          }
          frame "通道电压数" {
            w1561 = 2
            w1563 = FALSE
            n1110 = property on="从板个数" class="DigNum (严格)"("NumText.BGColor"=u32 13816530) -> ()  [unwired: 2 in, 2 out]
            n1111 = property on="电池实际容量(A)" class="DigNum (严格)"("Disabled"=w1561) -> ()  [unwired: 2 in, 2 out]
            n1112 = property on="使用者" class="DigNum (严格)"("Disabled"=w1561) -> ()  [unwired: 2 in, 2 out]
            n1113 = property on="SOH(%)" class="DigNum (严格)"("Disabled"=w1561) -> ()  [unwired: 2 in, 2 out]
            n1114 = property on="电池额定容量(A)" class="DigNum (严格)"("Disabled"=w1561) -> ()  [unwired: 2 in, 2 out]
            n1115 = property on="SOC(%)" class="DigNum (严格)"("Disabled"=w1561) -> ()  [unwired: 2 in, 2 out]
            n1116 = local read "从板个数"() -> (w1559:dbl)
            n1117 = property on="系统时钟" class="Str"("Disabled"=w1561) -> ()  [unwired: 2 in, 2 out]
            n1118 = property on="配置文件版本" class="Str"("Disabled"=w1561) -> ()  [unwired: 2 in, 2 out]
            n1119 = property on="车架(牌)号" class="Str"("Disabled"=w1561) -> ()  [unwired: 2 in, 2 out]
            n1120 = property on="产品编号" class="Str"("Disabled"=w1561) -> ()  [unwired: 2 in, 2 out]
            n1121 = control-ref of="项目信息"() -> (w1560:refnum<vi>)
            n1122 = stacked-sequence {
              tunnel: w1560 -> [w1570 w1573]
              tunnel: w1559 -> [w1569 w1572]
              frame #0 {
                n1123 = Compound Arithmetic op=ADD(1.0 ("值"), w1569) -> (w1566:dbl)
                n1124 = Bundle(w1566, 0) -> (w1568:cluster{dbl, i32})  [unwired: 1 out]
                n1125 = property class="Tbl (严格)"(reference=w1570, "Index Values"=w1568) -> ()  [unwired: 1 in, 2 out]
              }
              frame #1 {
                n1126 = for {
                  N: 20 -> [_]
                  tunnel: w1573 -> [w1581]
                  tunnel: w1572 -> [w1576]
                  i -> [w1575]
                  n1127 = Compound Arithmetic op=ADD(1.0 ("值"), w1576, w1575) -> (w1578:dbl)
                  n1128 = Bundle(w1578, 0) -> (w1580:cluster{dbl, i32})  [unwired: 1 out]
                  n1129 = property class="Tbl (严格)"(reference=w1581, "Active Cell"=w1580, "Cell BG Color"=u32 6618880) -> ()  [unwired: 1 in, 2 out]
                }
              }
            }
            n1130 = Select(t=0, s=w1549, f=1) -> (s? t:f=w1550:i32)
            n1131 = property on="项目信息" class="Tbl (严格)"("Disabled"=w1550) -> ()  [unwired: 2 in, 2 out]
            n1132 = global read "功能码全局.vi" "主板项目信息5"() -> (w1557:bool[])
            n1133 = global read "功能码全局.vi" "主板项目信息6"() -> (w1555:bool[])
            n1134 = Index Array(array=w1557, index=2 ("索引")) -> (element=w1554:bool)
            n1135 = Index Array(array=w1555, index=3 ("索引")) -> (element=w1553:bool)
            n1136 = Not(x=w1563) -> (.not. x?=w1562:bool)
          }
          frame "电压起始值" {
            w1595 = 2
            w1597 = FALSE
            n1137 = property on="从板个数" class="DigNum (严格)"("NumText.BGColor"=u32 13816530) -> ()  [unwired: 2 in, 2 out]
            n1138 = property on="电池实际容量(A)" class="DigNum (严格)"("Disabled"=w1595) -> ()  [unwired: 2 in, 2 out]
            n1139 = property on="使用者" class="DigNum (严格)"("Disabled"=w1595) -> ()  [unwired: 2 in, 2 out]
            n1140 = property on="SOH(%)" class="DigNum (严格)"("Disabled"=w1595) -> ()  [unwired: 2 in, 2 out]
            n1141 = property on="电池额定容量(A)" class="DigNum (严格)"("Disabled"=w1595) -> ()  [unwired: 2 in, 2 out]
            n1142 = property on="SOC(%)" class="DigNum (严格)"("Disabled"=w1595) -> ()  [unwired: 2 in, 2 out]
            n1143 = local read "从板个数"() -> (w1593:dbl)
            n1144 = property on="系统时钟" class="Str"("Disabled"=w1595) -> ()  [unwired: 2 in, 2 out]
            n1145 = property on="配置文件版本" class="Str"("Disabled"=w1595) -> ()  [unwired: 2 in, 2 out]
            n1146 = property on="车架(牌)号" class="Str"("Disabled"=w1595) -> ()  [unwired: 2 in, 2 out]
            n1147 = property on="产品编号" class="Str"("Disabled"=w1595) -> ()  [unwired: 2 in, 2 out]
            n1148 = control-ref of="项目信息"() -> (w1594:refnum<vi>)
            n1149 = stacked-sequence {
              tunnel: w1594 -> [w1604 w1607 w1620]
              tunnel: w1593 -> [w1603 w1606 w1619]
              frame #0 {
                n1150 = Compound Arithmetic op=ADD(21.0 ("值"), w1603) -> (w1600:dbl)
                n1151 = Bundle(w1600, 0) -> (w1602:cluster{dbl, i32})  [unwired: 1 out]
                n1152 = property class="Tbl (严格)"(reference=w1604, "Index Values"=w1602) -> ()  [unwired: 1 in, 2 out]
              }
              frame #1 {
                n1153 = for {
                  N: 10 -> [_]
                  tunnel: w1607 -> [w1617]
                  tunnel: w1606 -> [w1612]
                  i -> [w1611]
                  n1154 = Multiply(x=w1612, y=2.0) -> (x*y=w1609:dbl)
                  n1155 = Compound Arithmetic op=ADD(21.0 ("值"), w1609, w1611) -> (w1614:dbl)
                  n1156 = Bundle(w1614, 0) -> (w1616:cluster{dbl, i32})  [unwired: 1 out]
                  n1157 = property class="Tbl (严格)"(reference=w1617, "Active Cell"=w1616, "Cell BG Color"=u32 16448250) -> ()  [unwired: 1 in, 2 out]
                }
              }
              frame #2 {
                n1158 = Increment(x=w1619) -> (x+1=w1618:dbl)
                n1159 = for {
                  N: w1618 -> [_]
                  tunnel: w1620 -> [w1628]
                  tunnel: w1619 -> [w1623]
                  i -> [w1622]
                  n1160 = Compound Arithmetic op=ADD(21.0 ("值"), w1623, w1622) -> (w1625:dbl)
                  n1161 = Bundle(w1625, 0) -> (w1627:cluster{dbl, i32})  [unwired: 1 out]
                  n1162 = property class="Tbl (严格)"(reference=w1628, "Active Cell"=w1627, "Cell BG Color"=u32 6618880) -> ()  [unwired: 1 in, 2 out]
                }
              }
            }
            n1163 = Select(t=0, s=w1584, f=1) -> (s? t:f=w1583:i32)
            n1164 = property on="项目信息" class="Tbl (严格)"("Disabled"=w1583) -> ()  [unwired: 2 in, 2 out]
            n1165 = global read "功能码全局.vi" "主板项目信息5"() -> (w1591:bool[])
            n1166 = global read "功能码全局.vi" "主板项目信息6"() -> (w1589:bool[])
            n1167 = Index Array(array=w1591, index=3 ("索引")) -> (element=w1587:bool)
            n1168 = Index Array(array=w1589, index=4 ("索引")) -> (element=w1588:bool)
            n1169 = Not(x=w1597) -> (.not. x?=w1596:bool)
          }
          frame "温度个数" {
            w1642 = 2
            w1644 = FALSE
            n1170 = property on="电池实际容量(A)" class="DigNum (严格)"("Disabled"=w1642) -> ()  [unwired: 2 in, 2 out]
            n1171 = property on="使用者" class="DigNum (严格)"("Disabled"=w1642) -> ()  [unwired: 2 in, 2 out]
            n1172 = property on="SOH(%)" class="DigNum (严格)"("Disabled"=w1642) -> ()  [unwired: 2 in, 2 out]
            n1173 = property on="电池额定容量(A)" class="DigNum (严格)"("Disabled"=w1642) -> ()  [unwired: 2 in, 2 out]
            n1174 = property on="SOC(%)" class="DigNum (严格)"("Disabled"=w1642) -> ()  [unwired: 2 in, 2 out]
            n1175 = local read "从板个数"() -> (w1640:dbl)
            n1176 = control-ref of="项目信息"() -> (w1641:refnum<vi>)
            n1177 = stacked-sequence {
              tunnel: w1641 -> [w1649 w1652 w1659]
              tunnel: w1640 -> [w1646 w1651 w1658]
              frame #0 {
                n1178 = Bundle("从板个数"=w1646, 0) -> (w1648:cluster{"从板个数":dbl, i32})  [unwired: 1 out]
                n1179 = property class="Tbl (严格)"(reference=w1649, "Index Values"=w1648) -> ()  [unwired: 1 in, 2 out]
              }
              frame #1 {
                n1180 = for {
                  N: 20 -> [_]
                  tunnel: w1652 -> [w1657]
                  tunnel: w1651 -> [_]
                  i -> [w1653]
                  n1181 = Bundle(w1653, 0) -> (w1656:cluster{i32, i32})  [unwired: 1 out]
                  n1182 = property class="Tbl (严格)"(reference=w1657, "Active Cell"=w1656, "Cell BG Color"=u32 16448250) -> ()  [unwired: 1 in, 2 out]
                }
              }
              frame #2 {
                n1183 = for {
                  N: w1658 -> [_]
                  tunnel: w1659 -> [w1666]
                  tunnel: w1658 -> [w1660]
                  i -> [w1661]
                  n1184 = Compound Arithmetic op=ADD(w1660, w1661) -> (w1663:dbl)
                  n1185 = Bundle(w1663, 0) -> (w1665:cluster{dbl, i32})  [unwired: 1 out]
                  n1186 = property class="Tbl (严格)"(reference=w1666, "Active Cell"=w1665, "Cell BG Color"=u32 6618880) -> ()  [unwired: 1 in, 2 out]
                }
              }
            }
            n1187 = property on="系统时钟" class="Str"("Disabled"=w1642) -> ()  [unwired: 2 in, 2 out]
            n1188 = property on="配置文件版本" class="Str"("Disabled"=w1642) -> ()  [unwired: 2 in, 2 out]
            n1189 = property on="车架(牌)号" class="Str"("Disabled"=w1642) -> ()  [unwired: 2 in, 2 out]
            n1190 = property on="产品编号" class="Str"("Disabled"=w1642) -> ()  [unwired: 2 in, 2 out]
            n1191 = property on="从板个数" class="DigNum (严格)"("NumText.BGColor"=u32 13816530) -> ()  [unwired: 2 in, 2 out]
            n1192 = Select(t=0, s=w1631, f=1) -> (s? t:f=w1630:i32)
            n1193 = property on="项目信息" class="Tbl (严格)"("Disabled"=w1630) -> ()  [unwired: 2 in, 2 out]
            n1194 = global read "功能码全局.vi" "主板项目信息5"() -> (w1638:bool[])
            n1195 = global read "功能码全局.vi" "主板项目信息6"() -> (w1636:bool[])
            n1196 = Index Array(array=w1638, index=4 ("索引")) -> (element=w1634:bool)
            n1197 = Index Array(array=w1636, index=5 ("索引")) -> (element=w1635:bool)
            n1198 = Not(x=w1644) -> (.not. x?=w1643:bool)
          }
          frame "温度起始值" {
            w1680 = 2
            w1682 = FALSE
            n1199 = property on="电池实际容量(A)" class="DigNum (严格)"("Disabled"=w1680) -> ()  [unwired: 2 in, 2 out]
            n1200 = property on="使用者" class="DigNum (严格)"("Disabled"=w1680) -> ()  [unwired: 2 in, 2 out]
            n1201 = property on="SOH(%)" class="DigNum (严格)"("Disabled"=w1680) -> ()  [unwired: 2 in, 2 out]
            n1202 = property on="电池额定容量(A)" class="DigNum (严格)"("Disabled"=w1680) -> ()  [unwired: 2 in, 2 out]
            n1203 = property on="SOC(%)" class="DigNum (严格)"("Disabled"=w1680) -> ()  [unwired: 2 in, 2 out]
            n1204 = local read "从板个数"() -> (w1678:dbl)
            n1205 = property on="系统时钟" class="Str"("Disabled"=w1680) -> ()  [unwired: 2 in, 2 out]
            n1206 = property on="配置文件版本" class="Str"("Disabled"=w1680) -> ()  [unwired: 2 in, 2 out]
            n1207 = property on="车架(牌)号" class="Str"("Disabled"=w1680) -> ()  [unwired: 2 in, 2 out]
            n1208 = property on="产品编号" class="Str"("Disabled"=w1680) -> ()  [unwired: 2 in, 2 out]
            n1209 = control-ref of="项目信息"() -> (w1679:refnum<vi>)
            n1210 = stacked-sequence {
              tunnel: w1679 -> [w1691 w1694 w1707]
              tunnel: w1678 -> [w1684 w1693 w1706]
              frame #0 {
                n1211 = Multiply(x=w1684, y=3.0) -> (x*y=w1686:dbl)
                n1212 = Compound Arithmetic op=ADD(23.0 ("值"), w1686) -> (w1688:dbl)
                n1213 = Bundle(w1688, 0) -> (w1690:cluster{dbl, i32})  [unwired: 1 out]
                n1214 = property class="Tbl (严格)"(reference=w1691, "Index Values"=w1690) -> ()  [unwired: 1 in, 2 out]
              }
              frame #1 {
                n1215 = for {
                  N: 10 -> [_]
                  tunnel: w1694 -> [w1704]
                  tunnel: w1693 -> [w1699]
                  i -> [w1698]
                  n1216 = Multiply(x=4.0, y=w1699) -> (x*y=w1696:dbl)
                  n1217 = Compound Arithmetic op=ADD(24.0 ("值"), w1696, w1698) -> (w1701:dbl)
                  n1218 = Bundle(w1701, 0) -> (w1703:cluster{dbl, i32})  [unwired: 1 out]
                  n1219 = property class="Tbl (严格)"(reference=w1704, "Active Cell"=w1703, "Cell BG Color"=u32 16448250) -> ()  [unwired: 1 in, 2 out]
                }
              }
              frame #2 {
                n1220 = Increment(x=w1706) -> (x+1=w1705:dbl)
                n1221 = for {
                  N: w1705 -> [_]
                  tunnel: w1707 -> [w1717]
                  tunnel: w1706 -> [w1712]
                  i -> [w1711]
                  n1222 = Multiply(x=3.0, y=w1712) -> (x*y=w1709:dbl)
                  n1223 = Compound Arithmetic op=ADD(23.0 ("值"), w1709, w1711) -> (w1714:dbl)
                  n1224 = Bundle(w1714, 0) -> (w1716:cluster{dbl, i32})  [unwired: 1 out]
                  n1225 = property class="Tbl (严格)"(reference=w1717, "Active Cell"=w1716, "Cell BG Color"=u32 6618880) -> ()  [unwired: 1 in, 2 out]
                }
              }
            }
            n1226 = Select(t=0, s=w1669, f=1) -> (s? t:f=w1668:i32)
            n1227 = property on="从板个数" class="DigNum (严格)"("NumText.BGColor"=u32 13816530) -> ()  [unwired: 2 in, 2 out]
            n1228 = property on="项目信息" class="Tbl (严格)"("Disabled"=w1668) -> ()  [unwired: 2 in, 2 out]
            n1229 = global read "功能码全局.vi" "主板项目信息5"() -> (w1676:bool[])
            n1230 = global read "功能码全局.vi" "主板项目信息6"() -> (w1674:bool[])
            n1231 = Index Array(array=w1676, index=5 ("索引")) -> (element=w1673:bool)
            n1232 = Index Array(array=w1674, index=6 ("索引")) -> (element=w1672:bool)
            n1233 = Not(x=w1682) -> (.not. x?=w1681:bool)
          }
          frame "保险位置" {
            w1730 = 2
            w1732 = FALSE
            n1234 = property on="电池实际容量(A)" class="DigNum (严格)"("Disabled"=w1730) -> ()  [unwired: 2 in, 2 out]
            n1235 = property on="使用者" class="DigNum (严格)"("Disabled"=w1730) -> ()  [unwired: 2 in, 2 out]
            n1236 = property on="SOH(%)" class="DigNum (严格)"("Disabled"=w1730) -> ()  [unwired: 2 in, 2 out]
            n1237 = property on="电池额定容量(A)" class="DigNum (严格)"("Disabled"=w1730) -> ()  [unwired: 2 in, 2 out]
            n1238 = property on="SOC(%)" class="DigNum (严格)"("Disabled"=w1730) -> ()  [unwired: 2 in, 2 out]
            n1239 = local read "从板个数"() -> (w1728:dbl)
            n1240 = property on="系统时钟" class="Str"("Disabled"=w1730) -> ()  [unwired: 2 in, 2 out]
            n1241 = property on="配置文件版本" class="Str"("Disabled"=w1730) -> ()  [unwired: 2 in, 2 out]
            n1242 = property on="车架(牌)号" class="Str"("Disabled"=w1730) -> ()  [unwired: 2 in, 2 out]
            n1243 = property on="产品编号" class="Str"("Disabled"=w1730) -> ()  [unwired: 2 in, 2 out]
            n1244 = control-ref of="项目信息"() -> (w1729:refnum<vi>)
            n1245 = stacked-sequence {
              tunnel: w1729 -> [w1741 w1744]
              tunnel: w1728 -> [w1734 w1743]
              frame #0 {
                n1246 = Multiply(x=w1734, y=4.0) -> (x*y=w1736:dbl)
                n1247 = Compound Arithmetic op=ADD(24.0 ("值"), w1736) -> (w1738:dbl)
                n1248 = Bundle(w1738, 0) -> (w1740:cluster{dbl, i32})  [unwired: 1 out]
                n1249 = property class="Tbl (严格)"(reference=w1741, "Index Values"=w1740) -> ()  [unwired: 1 in, 2 out]
              }
              frame #1 {
                n1250 = for {
                  N: 20 -> [_]
                  tunnel: w1744 -> [w1754]
                  tunnel: w1743 -> [w1749]
                  i -> [w1748]
                  n1251 = Multiply(x=4.0, y=w1749) -> (x*y=w1746:dbl)
                  n1252 = Compound Arithmetic op=ADD(24.0 ("值"), w1746, w1748) -> (w1751:dbl)
                  n1253 = Bundle(w1751, 0) -> (w1753:cluster{dbl, i32})  [unwired: 1 out]
                  n1254 = property class="Tbl (严格)"(reference=w1754, "Active Cell"=w1753, "Cell BG Color"=u32 6618880) -> ()  [unwired: 1 in, 2 out]
                }
              }
            }
            n1255 = property on="从板个数" class="DigNum (严格)"("NumText.BGColor"=u32 13816530) -> ()  [unwired: 2 in, 2 out]
            n1256 = Select(t=0, s=w1721, f=1) -> (s? t:f=w1719:i32)
            n1257 = global read "功能码全局.vi" "主板项目信息4"() -> (w1726:bool[])
            n1258 = property on="项目信息" class="Tbl (严格)"("Disabled"=w1719) -> ()  [unwired: 2 in, 2 out]
            n1259 = Index Array(array=w1726, index #1=5 ("索引"), index #2=6 ("索引")) -> (element #1=w1724:bool, element #2=w1723:bool)
            n1260 = Not(x=w1732) -> (.not. x?=w1731:bool)
          }
          frame "SOC" {
            w1765 = 2
            w1767 = FALSE
            n1261 = property on="电池实际容量(A)" class="DigNum (严格)"("Disabled"=w1765) -> ()  [unwired: 2 in, 2 out]
            n1262 = property on="使用者" class="DigNum (严格)"("Disabled"=w1765) -> ()  [unwired: 2 in, 2 out]
            n1263 = property on="SOH(%)" class="DigNum (严格)"("Disabled"=w1765) -> ()  [unwired: 2 in, 2 out]
            n1264 = property on="电池额定容量(A)" class="DigNum (严格)"("Disabled"=w1765) -> ()  [unwired: 2 in, 2 out]
            n1265 = property on="从板个数" class="DigNum (严格)"("NumText.BGColor"=u32 13816530) -> ()  [unwired: 2 in, 2 out]
            n1266 = property on="系统时钟" class="Str"("Disabled"=w1765) -> ()  [unwired: 2 in, 2 out]
            n1267 = property on="配置文件版本" class="Str"("Disabled"=w1765) -> ()  [unwired: 2 in, 2 out]
            n1268 = property on="车架(牌)号" class="Str"("Disabled"=w1765) -> ()  [unwired: 2 in, 2 out]
            n1269 = property on="项目信息" class="Tbl (严格)"("Disabled"=w1765) -> ()  [unwired: 2 in, 2 out]
            n1270 = property on="产品编号" class="Str"("Disabled"=w1765) -> ()  [unwired: 2 in, 2 out]
            n1271 = Select(t=0, s=w1757, f=0) -> (s? t:f=w1756:i32)
            n1272 = property on="SOC(%)" class="DigNum (严格)"("Disabled"=w1756) -> ()  [unwired: 2 in, 2 out]
            n1273 = property on="项目信息2" class="Clust (严格)"("DisabledEnum"=w1756) -> ()  [unwired: 2 in, 2 out]
            n1274 = global read "功能码全局.vi" "主板项目信息7"() -> (w1763:bool[])
            n1275 = Index Array(array=w1763, index #1=2 ("索引"), index #2=5 ("索引")) -> (element #1=w1761:bool, element #2=w1760:bool)
            n1276 = Not(x=w1767) -> (.not. x?=w1766:bool)
          }
          frame "电池额定实际容量" {
            w1779 = 2
            w1781 = FALSE
            n1277 = property on="使用者" class="DigNum (严格)"("Disabled"=w1779) -> ()  [unwired: 2 in, 2 out]
            n1278 = property on="SOH(%)" class="DigNum (严格)"("Disabled"=w1779) -> ()  [unwired: 2 in, 2 out]
            n1279 = property on="SOC(%)" class="DigNum (严格)"("Disabled"=w1779) -> ()  [unwired: 2 in, 2 out]
            n1280 = property on="从板个数" class="DigNum (严格)"("NumText.BGColor"=u32 13816530) -> ()  [unwired: 2 in, 2 out]
            n1281 = property on="系统时钟" class="Str"("Disabled"=w1779) -> ()  [unwired: 2 in, 2 out]
            n1282 = property on="配置文件版本" class="Str"("Disabled"=w1779) -> ()  [unwired: 2 in, 2 out]
            n1283 = property on="车架(牌)号" class="Str"("Disabled"=w1779) -> ()  [unwired: 2 in, 2 out]
            n1284 = property on="项目信息" class="Tbl (严格)"("Disabled"=w1779) -> ()  [unwired: 2 in, 2 out]
            n1285 = property on="产品编号" class="Str"("Disabled"=w1779) -> ()  [unwired: 2 in, 2 out]
